vi "AO Reg UI.vi"(8 "error in (no error)":errorcluster, 11 "Node Ptr":T3 format="%.0x") -> (0 "error out":errorcluster)   [LabVIEW 2021, in "Modbus Master System Explorer.lvlib"]
uses:
  Modbus Master System Explorer.lvlib
  <vilib>/NI VeriStand/Custom Device API/Custom Device Item Ref.ctl
  Shared/Controls/Data Model/DataType.ctl
  SubVIs/Direction.ctl
  SubVIs/Modbus Type.ctl
  <vilib>/NI VeriStand/Custom Device API/Custom Device API.lvlib
  Shared/Modbus Master Shared.lvlib
panel:
  in  "Unit ID":u8
  in  "Default Value":dbl
  in  "Direction":T1
  out "Registers":i32
  in  "Sub-Index (Bool)":u16
  in  "DataType":T2
  in  "Valid?":string
  in  "Address":u16
  in  "Header":cluster{"Section Name":string}={"Section Name"="Holding Register (Analog Out) Settings"}
  in  "Description":string
  in  "Name":string
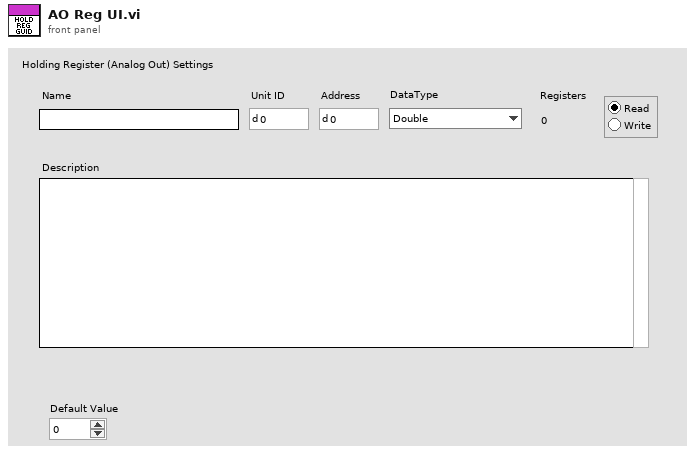
[diagram p1: front panel]
types:
  T1 = typedef "Modbus Master System Explorer.lvlib/Direction.ctl" = enum32{"Radio Selection 1", "Radio Selection 2"}
  T2 = typedef "Modbus Master Shared.lvlib/DataType.ctl" = enum16{"Double", "Single", "I64", "I32", "I16", "I8", "U64", "U32", "U16", "U8", "Boolean"}
  T3 = typedef "Custom Device API.lvlib/Custom Device Item Ref.ctl" = u64
  T4 = typedef "Modbus Master Shared.lvlib/Modbus Type.ctl" = enum16{"Coil", "Discrete Input", "Holding Register", "Input Register"}
  T5 = enum8{"Enabled", "Disabled", "Disabled and Grayed Out"}
  T6 = typedef "Custom Device API.lvlib/Custom Device Commands.ctl" = enum16{"Default", "Item renamed", "Shutdown", "Dynamic button pressed"}
  T7 = typedef "Custom Device API.lvlib/Custom Device Item Info.ctl" = cluster{"Name":string, "Is Channel":bool, "GUID":string, "Is Waveform":bool}
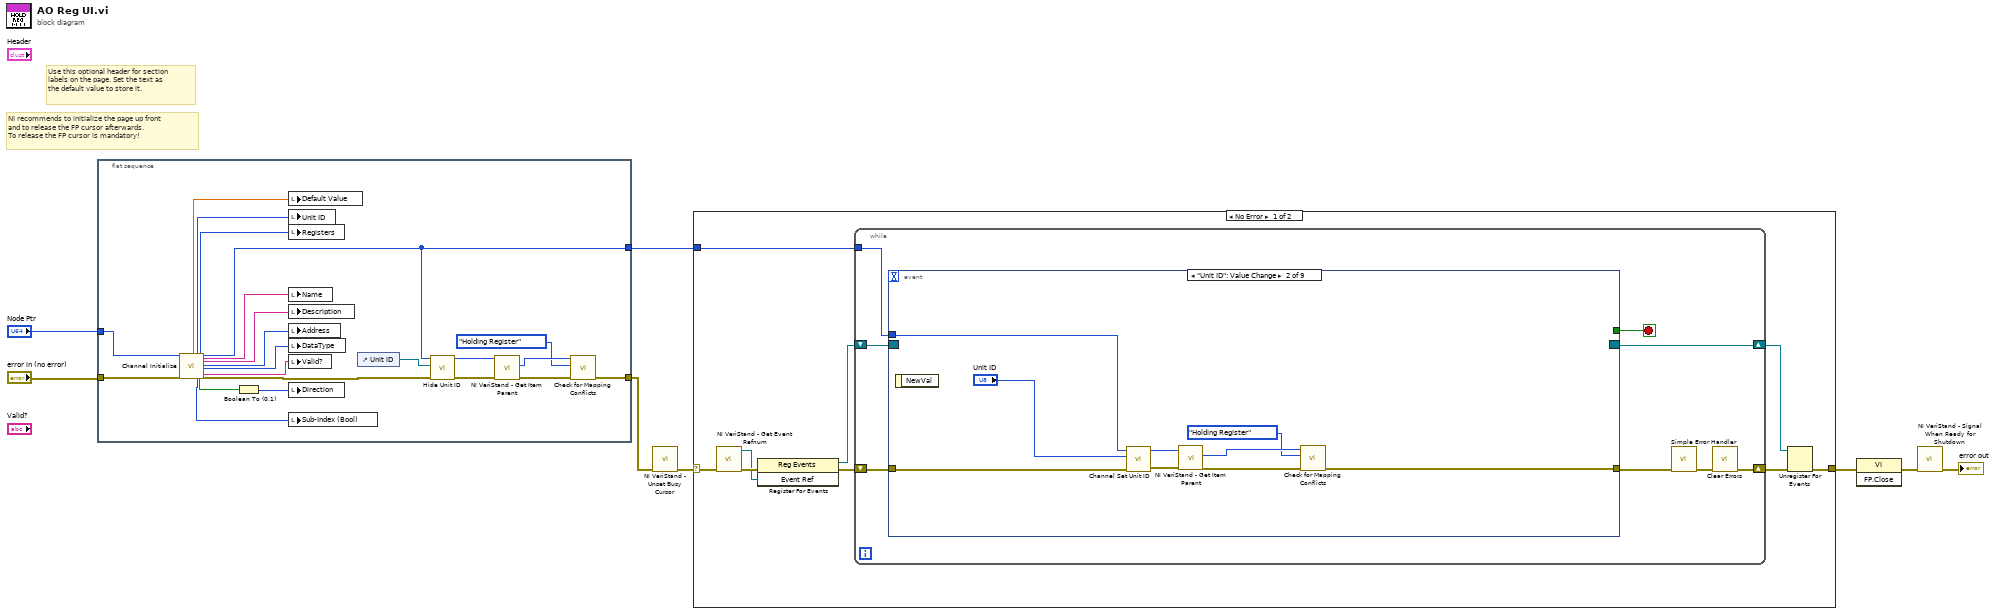
[diagram p0: block diagram]
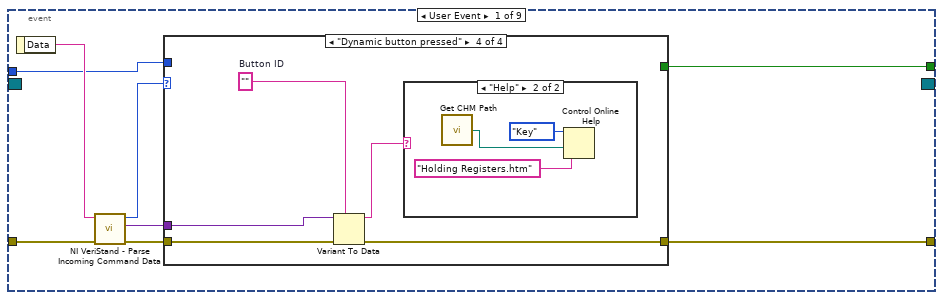
[diagram p2: hidden frame]
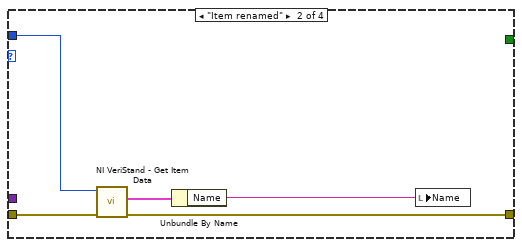
[diagram p4: hidden frame]
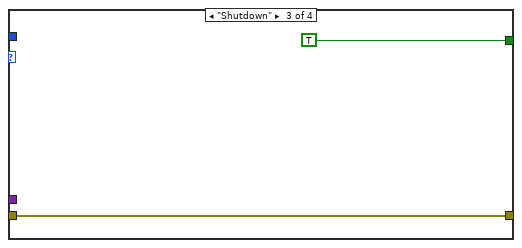
[diagram p5: hidden frame]
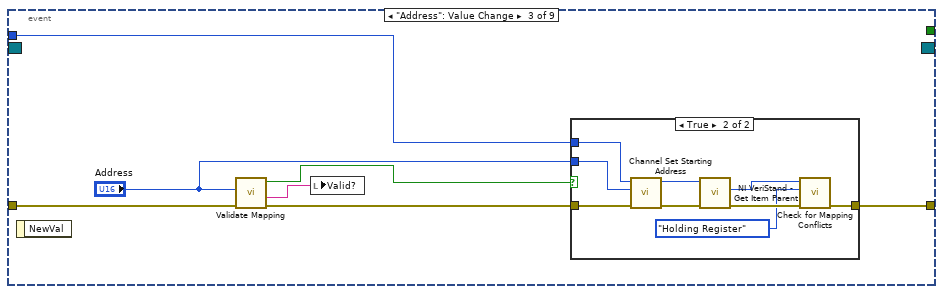
[diagram p7: hidden frame]
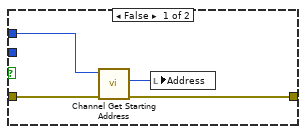
[diagram p8: hidden frame]
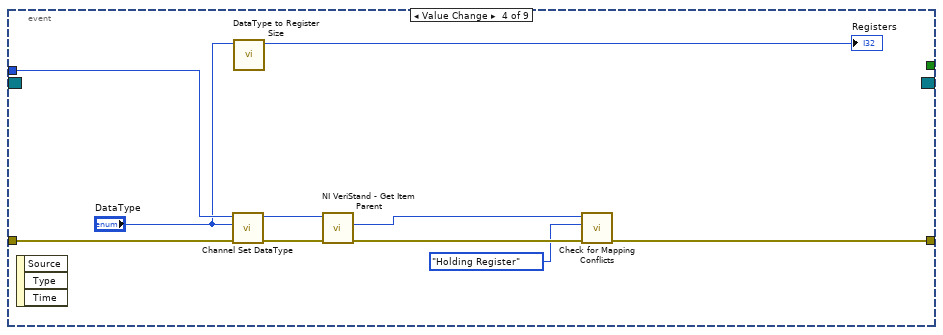
[diagram p9: hidden frame]
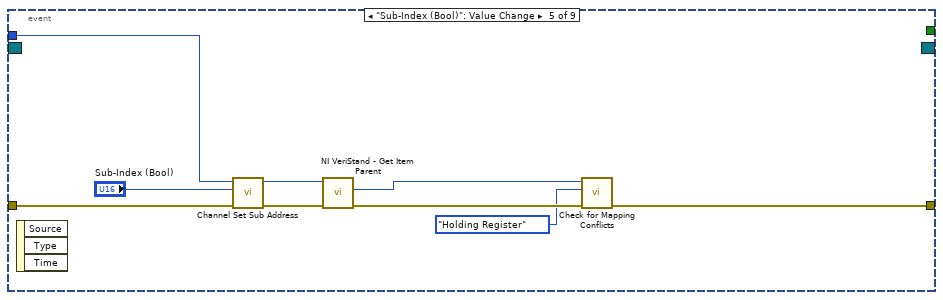
[diagram p10: hidden frame]
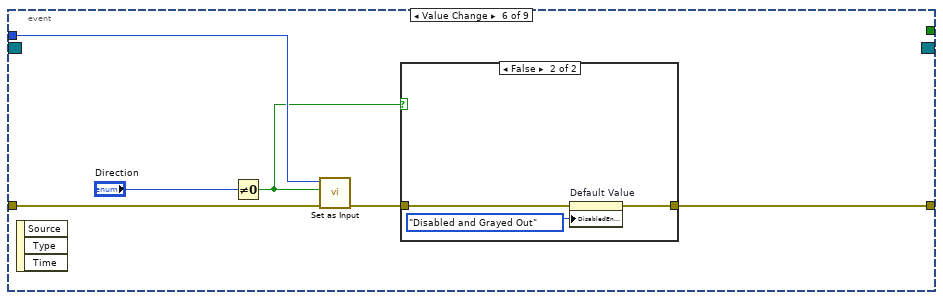
[diagram p11: hidden frame]
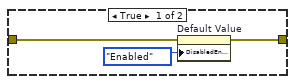
[diagram p12: hidden frame]
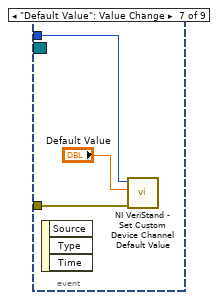
[diagram p13: hidden frame]
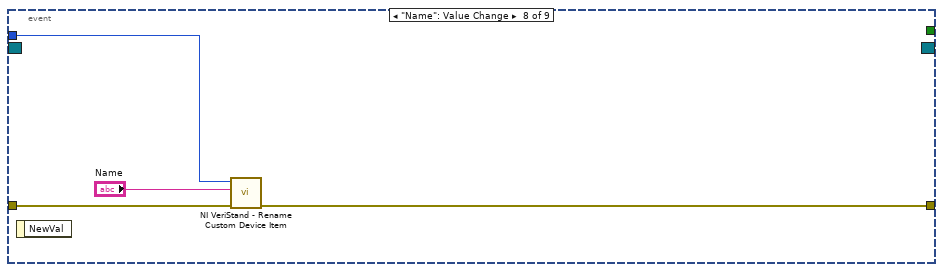
[diagram p14: hidden frame]
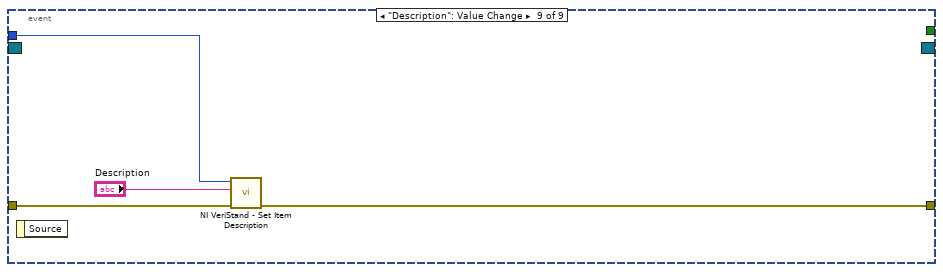
[diagram p15: hidden frame]
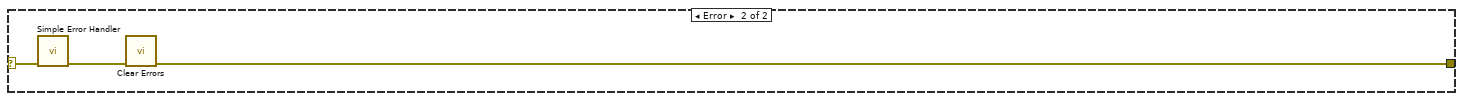
[diagram p16: hidden frame]
diagram:
  # "Use this optional header for section labels on the page. Set the text as the default value to store it."
  # "NI recommends to initialize the page up front\nand to release the FP cursor afterwards.\nTo release the FP cursor is mandatory!"
  n1 = flat-sequence {
    tunnel: "Node Ptr" -> [w21]
    tunnel: "error in (no error)" -> [w20]
    tunnel: [w11] -> w2
    tunnel: [w14] -> w1
    frame #0 {
      n2 = call "Channel Initialize.vi"("Item Ref in"=w21, "error in (no error)"=w20) -> ("Default Value"=w19:dbl, "Unit ID"=w18:u8, "Sub-Index (Bool)"=w25:u16, "Registers"=w26:i32, "input?"=w22:bool, "Channel Ref out"=w11:T3, "Name"=w29:string, "Description"=w30:string, "Starting Address"=w27:u16, "DataType"=w28:T2, "Status Message"=w24:string, "error out"=w10:errorcluster)  [unwired: 13 in, 1 out]
      n3 = Boolean To (0,1)(Boolean=w22) -> (0, 1=w23:i16)
      n4 = local write "Default Value"(w19) -> ()
      n5 = local write "Unit ID"(w18) -> ()
      n6 = local write "Registers"(w26) -> ()
      n7 = local write "Name"(w29) -> ()
      n8 = local write "Description"(w30) -> ()
      n9 = local write "Address"(w27) -> ()
      n10 = local write "DataType"(w28) -> ()
      n11 = local write "Valid?"(w24) -> ()
      n12 = local write "Direction"(w23) -> ()
      n13 = local write "Sub-Index (Bool)"(w25) -> ()
      n14 = control-ref of="Unit ID"() -> (w9:refnum<vi>)
      n15 = call "Hide Unit ID.vi"("error in (no error)"=w10, "Ctrl Ref"=w9, "Item Ref in"=w11) -> ("error out"=w12:errorcluster, "Item Ref out"=w13:T3)  [unwired: 7 in]
      n16 = call <vilib>:"NI VeriStand - Get Item Parent.vi"("error in (no error)"=w12, "Item Ref in"=w13) -> ("error out"=w15:errorcluster, "Parent Ref"=w17:T3)  [unwired: 6 in, 2 out]
      n17 = call "Check for Mapping Conflicts.vi"("error in (no error)"=w15, "Type"=Modbus_Type."Holding Register", "Coiil Group Ref in in"=w17) -> ("error out"=w14:errorcluster)  [unwired: 5 in, 3 out]
    }
  }
  n18 = call <vilib>:"NI VeriStand - Unset Busy Cursor.vi"("error in (no error)"=w1) -> ("error out"=w5:errorcluster)  [unwired: 10 out]
  n19 = case shown="No Error" w5 {
    selector: w5 -> [w31 w145]
    tunnel: [w36 w143] -> w8
    tunnel: w2 -> [w32 _]
    frame No Error {
      n20 = call <vilib>:"NI VeriStand - Get Event Refnum.vi"("error in (no error)"=w31) -> ("error out"=w39:errorcluster, "Event Ref"=w35:refnum<user-event>)  [unwired: 9 out]
      n21 = register-events(error in=w39, w35) -> (reference out=w33:refnum<event-registration>, error out=w34:errorcluster)  [unwired: 1 in]
      n22 = while {
        tunnel: w32 -> [w43]
        shift-right: [w40] -> w37
        shift-left: w34 -> [w46]
        shift-right: [w47] -> w38
        shift-left: w33 -> [w45]
        stop <- w44 stop-if-true
        n23 = event shown="[1] \"Unit ID\": Value Change" {
          selector: w45 -> [_ _ _ _ _ _ _ _ _]
          dyn-events: [_ _ _ _ _ _ _ _ _] -> w47
          timeout: _ -> [_ _ _ _ _ _ _ _ _]
          tunnel: w46 -> [w55 w80 w87 w110 w117 w124 w132 w138 w141]
          tunnel: [w51 _ _ _ _ _ _ _ _] -> w44
          tunnel: [w50 w72 w84 w104 w113 w121 _ w137 w140] -> w42
          tunnel: w43 -> [w49 w78 w86 w109 w119 w125 w133 w136 w142]
          event User Event {
            n24 = event-data() -> ("Data"=w54:string)  [unwired: 1 out]
            n25 = call <vilib>:"NI VeriStand - Parse Incoming Command Data.vi"("error in (no error)"=w55, "Incoming data"=w54) -> ("error out"=w53:errorcluster, "Outgoing data"=w48:variant, "Action"=w52:T6)  [unwired: 7 out]
            n26 = case shown="\"Dynamic button pressed\"" w52 {
              tunnel: w53 -> [w56 w61 w62 w68]
              tunnel: [_ _ TRUE _] -> w51
              tunnel: [w56 w58 w62 w65] -> w50
              tunnel: w49 -> [_ w60 _ _]
              tunnel: w48 -> [_ _ _ w67]
              frame "Default", Default {
              }
              frame "Item renamed" {
                n27 = call <vilib>:"NI VeriStand - Get Item Data.vi"("error in (no error)"=w61, "Item Ref in"=w60) -> ("error out"=w58:errorcluster, "Item Info"=w59:T7)  [unwired: 8 out]
                n28 = Unbundle By Name(w59) -> ("Name"=w57:string)
                n29 = local write "Name"(w57) -> ()
              }
              frame "Shutdown" {
              }
              frame "Dynamic button pressed" {
                w66 = ""  # Button ID
                n30 = Variant To Data(error in=w68, type=w66, Variant=w67) -> (data=w64:string, error out=w65:errorcluster)
                n31 = case shown="\"Help\"" w64 {
                  frame Default {
                  }
                  frame "Help" {
                    n32 = call "Get CHM Path.vi"() -> ("appended path"=w71:path)
                    n33 = Control Online Help(2:w71, 3:"Holding Registers.htm" ("String to search for"), 4:enum16{"Contents", "Key", "Close"}."Key" ("Operation")) -> ()  [unwired: 1 in, 1 out]
                  }
                }
              }
            }
          }
          event "Unit ID": Value Change {
            n34 = event-data() -> ()  [unwired: 2 out]
            n35 = call "Channel Set Unit ID.vi"("error in (no error)"=w80, "Value"="Unit ID", "Item Ref in"=w78) -> ("error out"=w73:errorcluster, "Item Ref out"=w74:T3)  [unwired: 7 in]
            n36 = call <vilib>:"NI VeriStand - Get Item Parent.vi"("error in (no error)"=w73, "Item Ref in"=w74) -> ("error out"=w76:errorcluster, "Parent Ref"=w77:T3)  [unwired: 6 in, 2 out]
            n37 = call "Check for Mapping Conflicts.vi"("error in (no error)"=w76, "Type"=Modbus_Type."Holding Register", "Coiil Group Ref in in"=w77) -> ("error out"=w72:errorcluster)  [unwired: 5 in, 3 out]
          }
          event "Address": Value Change {
            n38 = event-data() -> ()  [unwired: 2 out]
            n39 = call "Validate Mapping.vi"("error in (no error)"=w87, "Mapping"="Address") -> ("error out"=w85:errorcluster, "Status Message"=w81:string, "Valid?"=w83:bool)  [unwired: 7 in]
            n40 = local write "Valid?"(w81) -> ()
            n41 = case shown="True" w83 {
              tunnel: w86 -> [w91 w99]
              tunnel: w85 -> [w90 w100]
              tunnel: [w89 w93] -> w84
              tunnel: "Address" -> [_ w98]
              frame False {
                n42 = call "Channel Get Starting Address.vi"("error in (no error)"=w90, "Item Ref in"=w91) -> ("error out"=w89:errorcluster, "Value"=w88:u16)  [unwired: 7 in, 1 out]
                n43 = local write "Address"(w88) -> ()
              }
              frame True {
                n44 = call "Channel Set Starting Address.vi"("error in (no error)"=w100, "Value"=w98, "Item Ref in"=w99) -> ("error out"=w97:errorcluster, "Item Ref out"=w96:T3)  [unwired: 7 in]
                n45 = call <vilib>:"NI VeriStand - Get Item Parent.vi"("error in (no error)"=w97, "Item Ref in"=w96) -> ("error out"=w94:errorcluster, "Parent Ref"=w95:T3)  [unwired: 6 in, 2 out]
                n46 = call "Check for Mapping Conflicts.vi"("error in (no error)"=w94, "Type"=Modbus_Type."Holding Register", "Coiil Group Ref in in"=w95) -> ("error out"=w93:errorcluster)  [unwired: 5 in, 3 out]
              }
            }
          }
          event Value Change {
            n47 = event-data() -> ()  [unwired: 4 out]
            n48 = call "Channel Set DataType.vi"("error in (no error)"=w110, "DataType"="DataType", "Item Ref in"=w109) -> ("error out"=w105:errorcluster, "Item Ref out"=w107:T3)  [unwired: 7 in]
            n49 = call "DataType to Register Size.vi"("DataType"="DataType") -> ("Registers"=→"Registers":i32)  [unwired: 9 in, 1 out]
            n50 = call <vilib>:"NI VeriStand - Get Item Parent.vi"("error in (no error)"=w105, "Item Ref in"=w107) -> ("error out"=w106:errorcluster, "Parent Ref"=w108:T3)  [unwired: 6 in, 2 out]
            n51 = call "Check for Mapping Conflicts.vi"("error in (no error)"=w106, "Type"=Modbus_Type."Holding Register", "Coiil Group Ref in in"=w108) -> ("error out"=w104:errorcluster)  [unwired: 5 in, 3 out]
          }
          event "Sub-Index (Bool)": Value Change {
            n52 = event-data() -> ()  [unwired: 4 out]
            n53 = call "Channel Set Sub Address.vi"("error in (no error)"=w117, "Value"="Sub-Index (Bool)", "Item Ref in"=w119) -> ("error out"=w115:errorcluster, "Item Ref out"=w112:T3)  [unwired: 7 in]
            n54 = call <vilib>:"NI VeriStand - Get Item Parent.vi"("error in (no error)"=w115, "Item Ref in"=w112) -> ("error out"=w114:errorcluster, "Parent Ref"=w116:T3)  [unwired: 6 in, 2 out]
            n55 = call "Check for Mapping Conflicts.vi"("error in (no error)"=w114, "Type"=Modbus_Type."Holding Register", "Coiil Group Ref in in"=w116) -> ("error out"=w113:errorcluster)  [unwired: 5 in, 3 out]
          }
          event Value Change {
            n56 = event-data() -> ()  [unwired: 4 out]
            n57 = Not Equal To 0?(x="Direction") -> (x != 0?=w120:bool)
            n58 = call "Set as Input.vi"("error in (no error)"=w124, "Direction"=w120, "Channel Ref in"=w125) -> ("error out"=w122:errorcluster)  [unwired: 7 in, 1 out]
            n59 = case shown="False" w120 {
              tunnel: w122 -> [w127 w130]
              tunnel: [w126 w129] -> w121
              frame True {
                n60 = property on="Default Value" class="DigNum (strict)"(error in=w127, "DisabledEnum"=T5."Enabled" ("Disabled")) -> (error out=w126:errorcluster)  [unwired: 1 in, 1 out]
              }
              frame False {
                n61 = property on="Default Value" class="DigNum (strict)"(error in=w130, "DisabledEnum"=T5."Disabled and Grayed Out" ("Disabled")) -> (error out=w129:errorcluster)  [unwired: 1 in, 1 out]
              }
            }
          }
          event "Default Value": Value Change {
            n62 = event-data() -> ()  [unwired: 4 out]
            n63 = call <vilib>:"NI VeriStand - Set Custom Device Channel Default Value.vi"("error in (no error)"=w132, "Default Value"="Default Value", "Channel Ref in"=w133) -> ()  [unwired: 7 in, 2 out]
          }
          event "Name": Value Change {
            n64 = event-data() -> ()  [unwired: 2 out]
            n65 = call <vilib>:"NI VeriStand - Rename Custom Device Item.vi"("error in (no error)"=w138, "New Name"="Name", "Item Ref in"=w136) -> ("error out"=w137:errorcluster)  [unwired: 1 in, 7 out]
          }
          event "Description": Value Change {
            n66 = event-data() -> ()  [unwired: 2 out]
            n67 = call <vilib>:"NI VeriStand - Set Item Description.vi"("error in (no error)"=w141, "Description"="Description", "Item Ref in"=w142) -> ("error out"=w140:errorcluster)  [unwired: 8 out]
          }
        }
        n68 = call <vilib>:"Simple Error Handler.vi"("error in (no error)"=w42) -> ("error out"=w41:errorcluster)  [unwired: 1 in, 7 out]
        n69 = call <vilib>:"Clear Errors.vi"("error in (no error)"=w41) -> ("error out"=w40:errorcluster)  [unwired: 1 in, 5 out]
      }
      n70 = Unregister For Events(event registration refnum=w38, error in=w37) -> (error out=w36:errorcluster)
    }
    frame Error {
      n71 = call <vilib>:"Simple Error Handler.vi"("error in (no error)"=w145) -> ("error out"=w144:errorcluster)  [unwired: 1 in, 7 out]
      n72 = call <vilib>:"Clear Errors.vi"("error in (no error)"=w144) -> ("error out"=w143:errorcluster)  [unwired: 1 in, 5 out]
    }
  }
  n73 = invoke class="VI" method="FP.Close"(error in=w8) -> (error out=w7:errorcluster)  [unwired: 2 in, 2 out]
  n74 = call <vilib>:"NI VeriStand - Signal When Ready for Shutdown.vi"("error in (no error)"=w7) -> ("error out"=→"error out":errorcluster)  [unwired: 10 out]
